vi "ReportInitDone.vi"(2 "error in (no error)":errorcluster, 3 "Preferences in":refnum<class "SetListPrefs.lvclass">) -> (0 "error out":errorcluster, 1 "Preferences out":refnum<class "SetListPrefs.lvclass">)   [LabVIEW 2013, in "SetListPrefs.lvclass"]
uses:
  SetListPrefs.lvclass
  SetListPrefs.lvclass/SetListPrefs.ctl
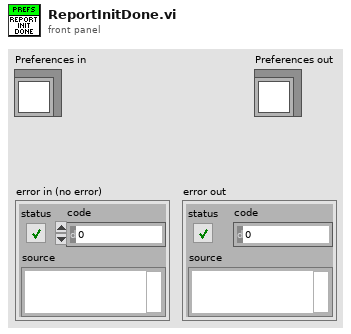
[diagram p1: front panel]
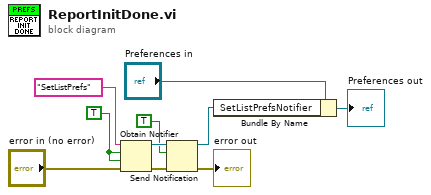
[diagram p0: block diagram]
diagram:
  w7 = TRUE
  n1 = Obtain Notifier(name (unnamed)="SetListPrefs", notification data type=w7, create if not found? (T)=w7, error in (no error)="error in (no error)") -> (notifier out=w9:refnum<notifier>, error out=w10:errorcluster)  [unwired: 1 out]
  n2 = Send Notification(notification=TRUE, notifier=w9, error in (no error)=w10) -> (notifier out=w2:refnum<notifier>, error out=→"error out":errorcluster)
  n3 = Bundle By Name(cluster="Preferences in", "SetListPrefsNotifier"=w2) -> (→"Preferences out":refnum<class "SetListPrefs.lvclass">)
